vi "host-C_Exp.vi"() -> (0 "K(Indicator)":fxp<+/-,64,32>=1.52587890625e-05, 1 "degree":dbl=0.1952712924057206, 2 "Nominal Freq":fxp<+/-,64,32>=0.494873046875)   [LabVIEW 2012]
uses:
  <vilib>/FPGAPlugInAG/PCI-7831R/niLvFpga_Open_PCI-7831R.vi
  <vilib>/Utility/error.llb/Error Cluster From Error Code.vi
  <vilib>/rvi/errors/niLvFpgaAdjustHostInterfaceError.vi
  <vilib>/FPGAPlugInAG/PCI-7831R/niLvFpga_Run_PCI-7831R.vi
  <vilib>/FPGAPlugInAG/PCI-7831R/niLvFpga_Abort_PCI-7831R.vi
  <vilib>/FPGAPlugInAG/PCI-7831R/niLvFpga_Close_PCI-7831R.vi
  <vilib>/rvi/interface/common/dynamic/niFpgaDynamicAddResources.vi
  <vilib>/FPGAPlugInAG/Dynamic/niLvFpga_Abort_Dynamic.vi
  <vilib>/FPGAPlugInAG/Dynamic/niLvFpga_Close_Dynamic.vi
  <vilib>/Utility/file.llb/Write To Spreadsheet File (DBL).vi
  <vilib>/rvi/interface/nirviOpenFPGA/nirviOpenFPGA.xnode
  SB130-XPS/Documents/FPGA-project-apporach-retraction/FPGA Bitfiles/Apporach-Retract_FPGATarget_LIAFPGA3a-PDTest_L-X5ia9B-g4.lvbitx
  LIA_FPGA3a-PD Test.vi
  <vilib>/rvi/interface/nirviReadWriteControl/nirviReadWriteControl.xnode
  <vilib>/rvi/interface/nirviMethod/nirviMethod.xnode
  <vilib>/rvi/interface/nirviCloseFPGA/nirviCloseFPGA.xnode
  NiFpgaLv.dll
  <vilib>/rvi/interface/Simulation/niFpgaSimulationCallBeginRW.vi
panel:
  in  "Path 5":path
  in  "name-file 11":string="approach-15a"
  out "String 11":string
  in  "Path 7":path
  in  "name-file 9":string="approach-15a"
  out "String 9":string
  out "P+I Error":dbl
  in  "Integral Gain":dbl
  in  "Proportional Gain":ext
  out "Setpoint":dbl
  in  "Path 4":path
  in  "name-file 4":string="approach-15a"
  out "String 4":string
  in  "Path 3":path
  in  "name-file 3":string="approach-15a"
  out "String 3":string
  in  "Path 2":path
  in  "name-file 2":string="approach-15a"
  out "String 2":string
  in  "Data Collector":bool
  out "String":string
  in  "name-file":string="approach-15a"
  in  "Path":path
  out "Standardized nominal freq":dbl
  in  "Delta Nominal Frequency":dbl
  out "Ref":i32
  out "Sig":i32
  out "Sin":dbl(graph)
  out "Phase":dbl
  out "Ze Output":dbl=2.3841857910156248e-12
  out "The Decs":dbl=7.8125e-09
  out "LSB Weight":dbl=0.00030517578125
  in  "K":fxp<+,16,0>=1.52587890625e-05
  in  "nominal freq 2":fxp<+,16,0>=0.494873046875
  out "x*y":dbl=0.015
  in  "stop 2":bool
  out "3rd stages":i32=1
  out "3rd decimation":i32=977
  out "1st decimation":i32=1
  out "2nd decimation":i32=128
  in  "Time Constant [s]":dbl=2.5 min=0.0 step=0.0001 format="%.2f"
  in  "Filter Rolloff":enum16{"20 dB", "40 dB", "60 dB", "80 dB"}(ring)
  out "Actual Sampling Frequency":dbl=200000.0
  in  "input range of 9205":dbl=10.0
  in  "Sampling Frequency":dbl=200000.0 min=1000.0 max=250000.0
  in  "stop":bool
  out "r":dbl(graph)=0.5098420210496609
  out "y":dbl=0.0017376029872894286
  out "x":dbl=0.5098390600609779
  out "f":dbl(graph)=31000.332441180944
  in  "dec2":i16=1
  in  "nominal freq":dbl=30000.0 min=500.0 max=125000.0
  in  "dec1":i16=1000
  in  "stages":i8=1 min=1 max=2
  in  "decimation":i16=1000
  # "Sampling Frequency"
  # "CIC First Decimation"
  # "MA Stages"
  # "CIC Second Decimation"
  # "PLL Nominal Frequency"
  # "MA Decimation"
  # "PLL Frequency Output"
  # "LIA Output"
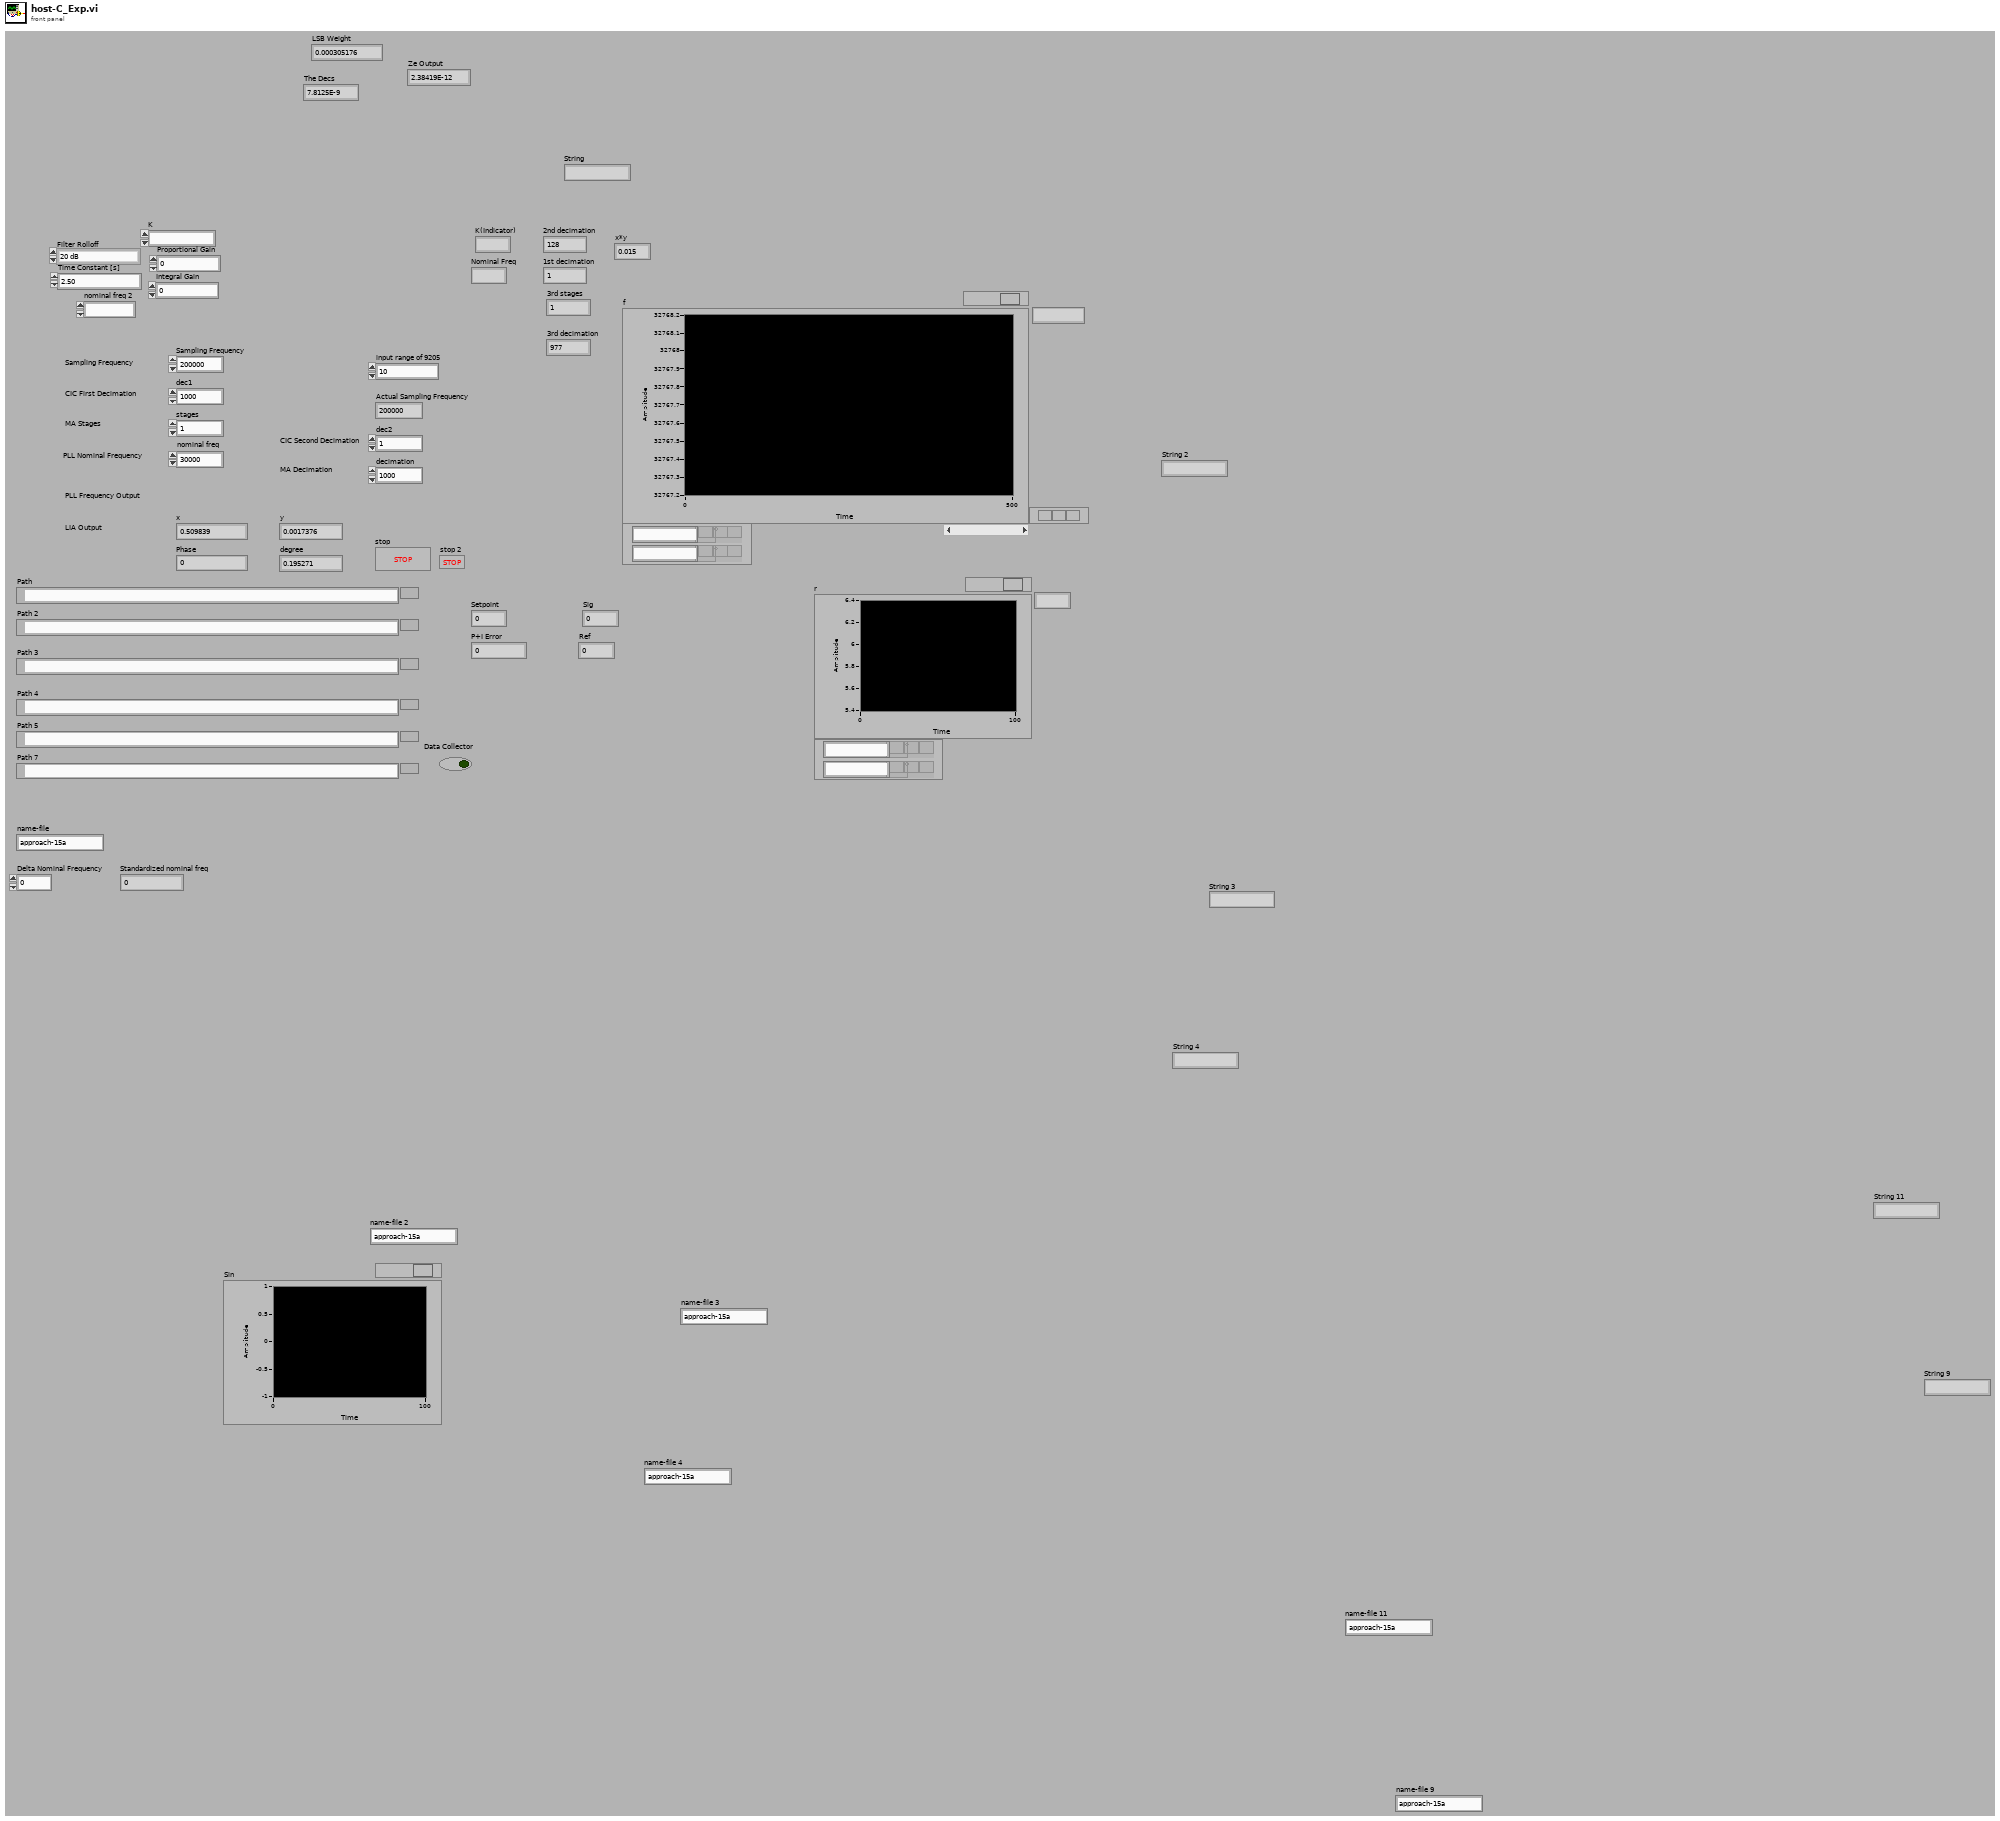
[diagram p1: front panel]
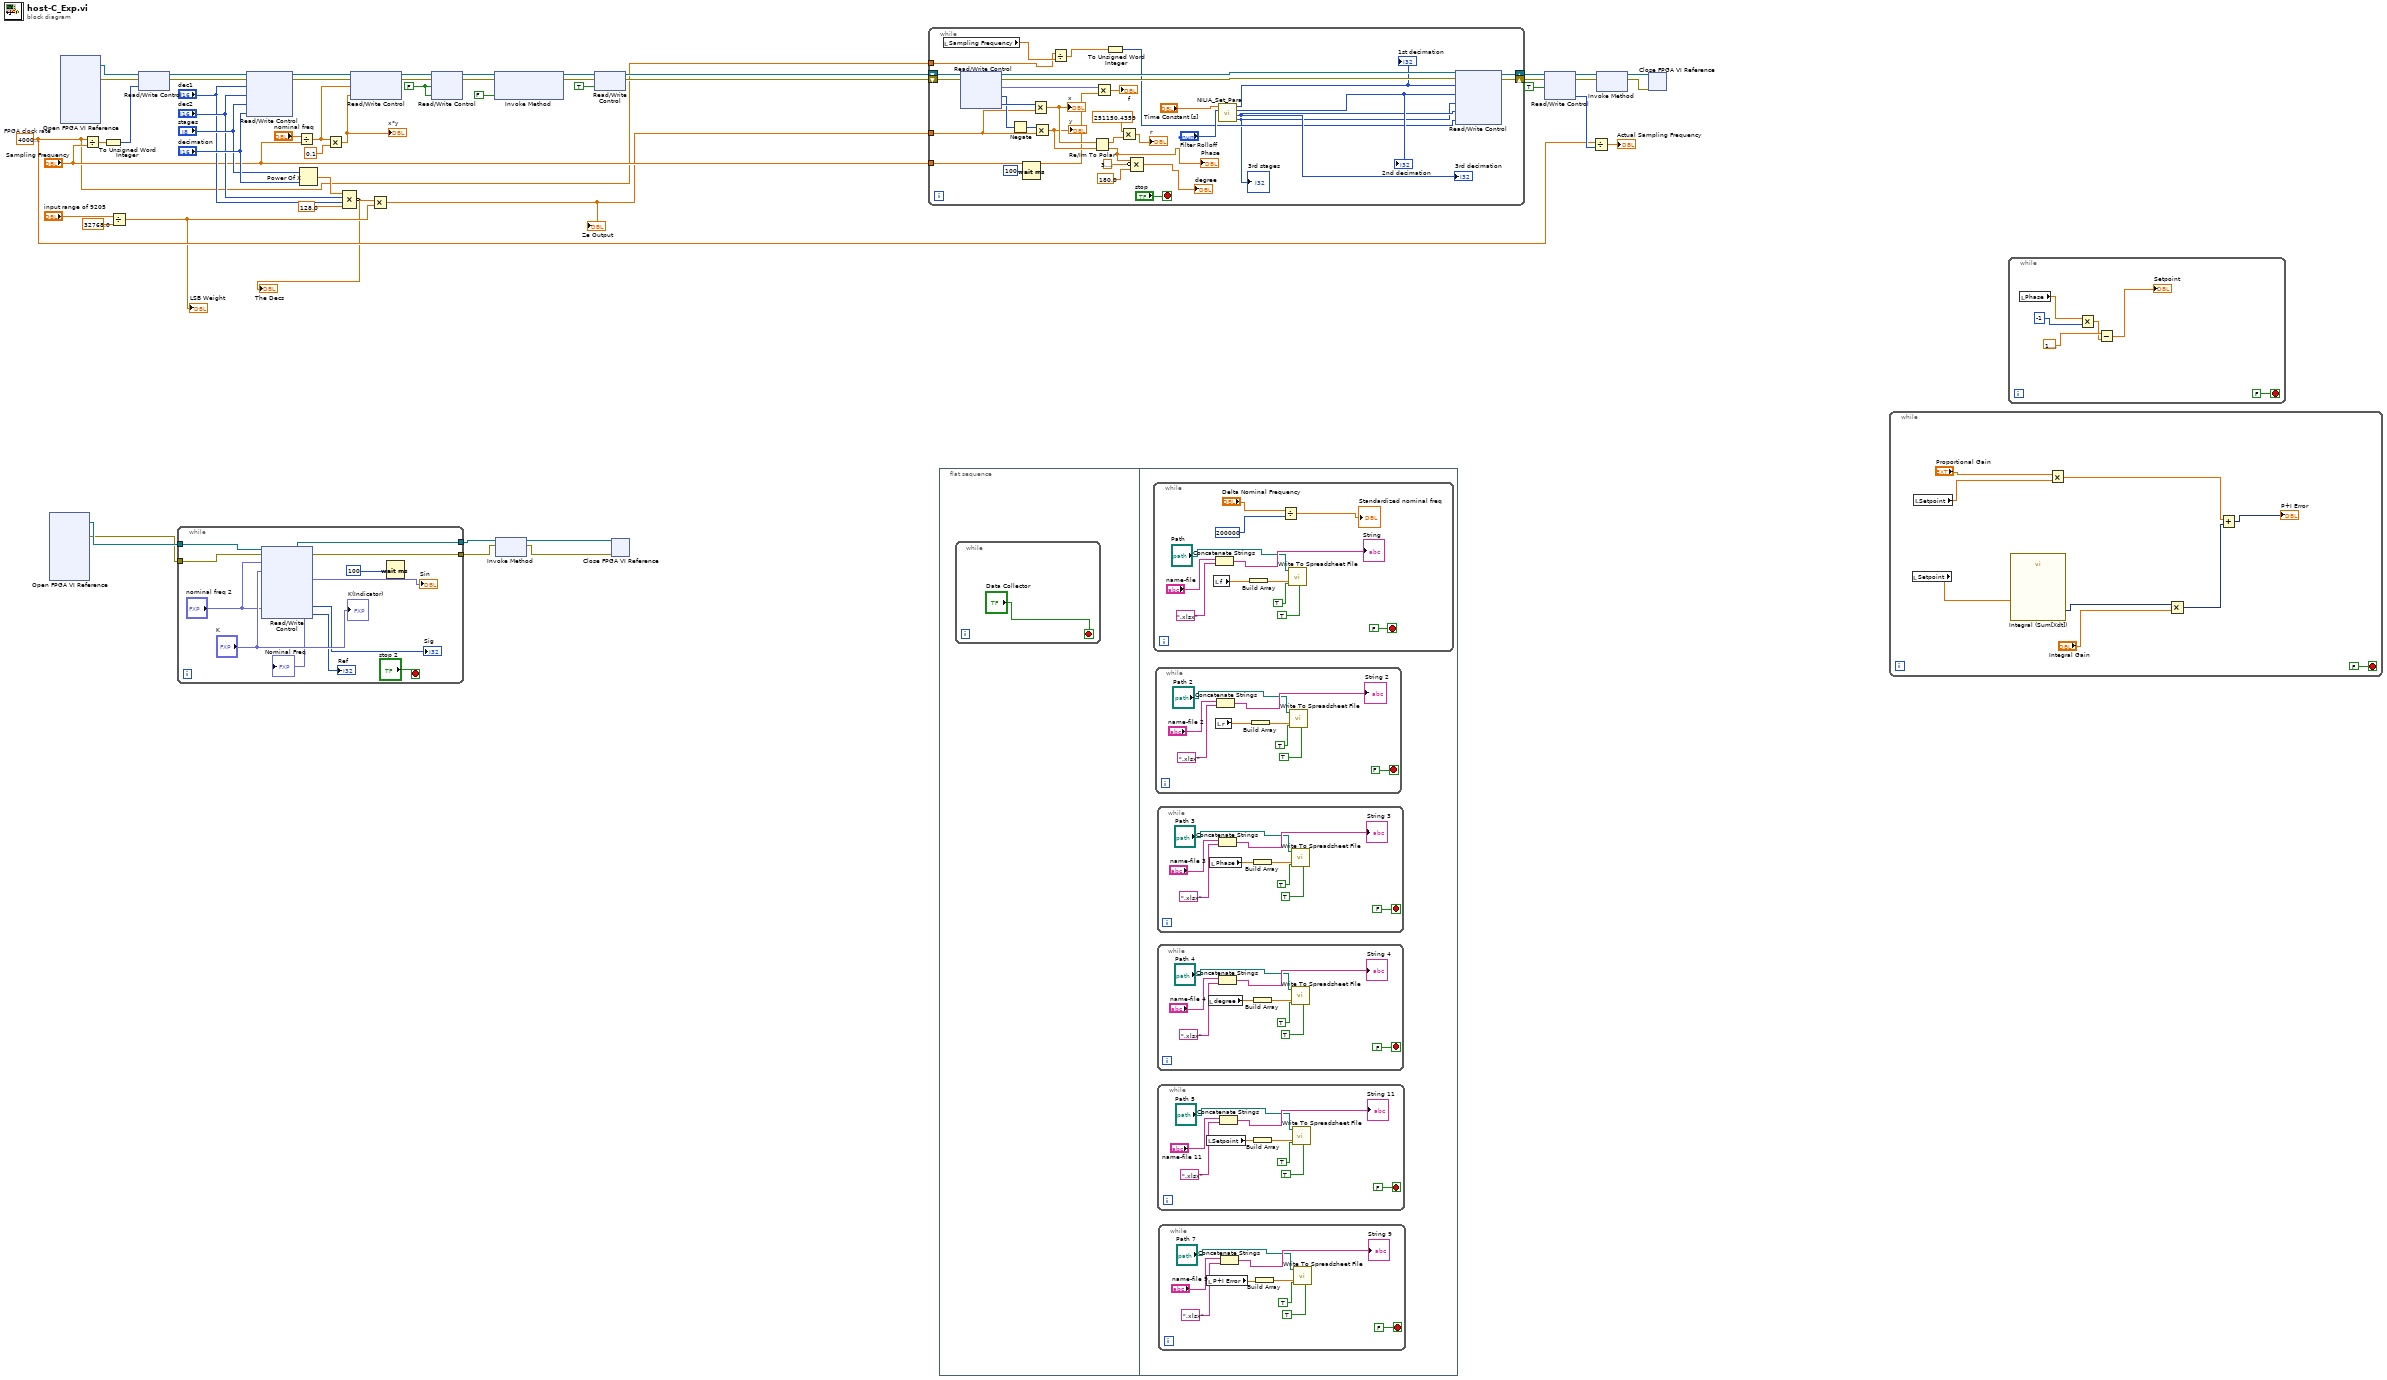
[diagram p0: block diagram]
diagram:
  w13 = 40000000.0  # FPGA clock rate
  w30 = FALSE ("start")
  n1 = xnode "Open FPGA VI Reference"() -> ("FPGA VI Reference Out"=w2:refnum<k20>, "error out"=w1:errorcluster)  [unwired: 2 in]
  n2 = xnode "Open FPGA VI Reference"() -> ("FPGA VI Reference Out"=w3:refnum<k20>, "error out"=w4:errorcluster)  [unwired: 2 in]
  n3 = Divide(x=w13, y="Sampling Frequency") -> (x/y=w23:dbl)
  n4 = To Unsigned Word Integer(number=w23) -> (unsigned 16bit integer=w22:u16)
  n5 = Divide(x="input range of 9205", y=32768.0) -> (x/y=w7:dbl)
  "LSB Weight" <- w7
  n6 = xnode "Read/Write Control"("FPGA VI Reference In"=w3, "error in"=w4, "Period"=w22) -> ("FPGA VI Reference Out"=w25:refnum<k20>, "error out"=w24:errorcluster)
  n7 = while {
    tunnel: w2 -> [w52]
    tunnel: w1 -> [w61]
    tunnel: [w60] -> w12
    tunnel: [w59] -> w11
    stop <- "stop 2" stop-if-true
    n8 = xnode "Read/Write Control"("FPGA VI Reference In"=w52, "error in"=w61, "nominal freq"="nominal freq 2", "K"="K") -> ("FPGA VI Reference Out"=w60:refnum<k20>, "error out"=w59:errorcluster, "Sin"=→"Sin":fxp<+/-,14,2>, "sig"=→"Sig":i16, "ref"=→"Ref":i16)  [unwired: 2 out]
    n9 = Wait (ms)(milliseconds to wait=u32 100) -> ()  [unwired: 1 out]
    "K(Indicator)" <- "K"
    "Nominal Freq" <- "nominal freq 2"
  }
  n10 = xnode "Read/Write Control"("FPGA VI Reference In"=w25, "error in"=w24, "dec1"="dec1", "dec2"="dec2", "stages"="stages", "decimation"="decimation") -> ("FPGA VI Reference Out"=w51:refnum<k20>, "error out"=w50:errorcluster)
  n11 = Divide(x="nominal freq", y="Sampling Frequency") -> (x/y=w19:dbl)
  n12 = Power Of X(1:"decimation", 2:"stages") -> (0:w46:dbl)
  n13 = Multiply(x=w19, y=0.1) -> (x*y=w8:dbl)
  "x*y" <- w8
  n14 = Compound Arithmetic op=MULTIPLY(w46, "dec2", "dec1", 128.0) -> (invert w6:dbl)
  "The Decs" <- w6
  n15 = xnode "Read/Write Control"("FPGA VI Reference In"=w51, "error in"=w50, "nominal freq"=w19, "K"=w8) -> ("FPGA VI Reference Out"=w34:refnum<k20>, "error out"=w33:errorcluster)
  n16 = Multiply(x=w6, y=w7) -> (x*y=w5:dbl)
  "Ze Output" <- w5
  n17 = xnode "Read/Write Control"("FPGA VI Reference In"=w34, "error in"=w33, "start"=w30, "stop"=w30) -> ("FPGA VI Reference Out"=w32:refnum<k20>, "error out"=w31:errorcluster)
  n18 = xnode "Invoke Method"("FPGA VI Reference In"=w32, "error in"=w31, "Wait Until Done (F)"=FALSE) -> ("FPGA VI Reference Out"=w39:refnum<k20>, "error out"=w37:errorcluster)
  n19 = xnode "Invoke Method"("FPGA VI Reference In"=w12, "error in"=w11) -> ("FPGA VI Reference Out"=w10:refnum<k20>, "error out"=w9:errorcluster)
  n20 = xnode "Read/Write Control"("FPGA VI Reference In"=w39, "error in"=w37, "start"=TRUE) -> ("FPGA VI Reference Out"=w38:refnum<k20>, "error out"=w36:errorcluster)
  n21 = xnode "Close FPGA VI Reference"("FPGA VI Reference In"=w10, "error in"=w9) -> ()  [unwired: 1 out]
  n22 = while {
    shift-right: [w79] -> w42
    shift-left: w38 -> [w94]
    shift-right: [w78] -> w41
    shift-left: w36 -> [w93]
    tunnel: w5 -> [w90]
    tunnel: "Sampling Frequency" -> [w82]
    tunnel: w13 -> [w71]
    stop <- "stop" stop-if-true
    n23 = local read "Sampling Frequency"() -> (w72:dbl)
    n24 = xnode "Read/Write Control"("FPGA VI Reference In"=w94, "error in"=w93) -> ("FPGA VI Reference Out"=w79:refnum<k20>, "error out"=w78:errorcluster, "f"=w83:fxp<+/-,32,0>, "channelQ"=w91:i64, "channelI"=w92:i64)
    n25 = Negate(x=w91) -> (-x=w80:i64)
    n26 = Wait (ms)(milliseconds to wait=u32 100) -> ()  [unwired: 1 out]
    n27 = Multiply(x=w92, y=w90) -> (x*y=w89:dbl)
    "x" <- w89
    n28 = Multiply(x=w80, y=w90) -> (x*y=w88:dbl)
    "y" <- w88
    n29 = Divide(x=w71, y=w72) -> (x/y=w70:dbl)
    n30 = Re/Im To Polar(2:w88, 3:w89) -> (0:w63:dbl, 1:w66:dbl)
    "Phase" <- w63
    n31 = Multiply(x=w83, y=w82) -> (x*y=→"f":dbl)
    n32 = To Unsigned Word Integer(number=w70) -> (unsigned 16bit integer=w69:u16)
    n33 = Multiply(x=251150.4359, y=w66) -> (x*y=→"r":dbl)
    n34 = Compound Arithmetic op=MULTIPLY(w63, invert 3.141592653589793, 180.0 ("value")) -> (→"degree":dbl)
    n35 = call "NILIA_Set_Para.vi"("rolloff"="Filter Rolloff", "TC [sec]"="Time Constant [s]") -> ("3rd stages"=w68:i32, "3rd decimation"=w73:i32, "2nd decimation"=w74:i32, "1st decimation"=w75:i32)  [unwired: 5 in, 1 out]
    "2nd decimation" <- w74
    "1st decimation" <- w75
    "3rd decimation" <- w73
    "3rd stages" <- w68
    n36 = xnode "Read/Write Control"("FPGA VI Reference In"=w79, "error in"=w78, "dec1"=w75, "dec2"=w74, "stages"=w68, "decimation"=w73, "Period"=w69) -> ()  [unwired: 2 out]
  }
  n37 = flat-sequence {
    frame #0 {
      n38 = while {
        stop <- "Data Collector" stop-if-true
      }
    }
    frame #1 {
      n39 = while {
        stop <- FALSE stop-if-true
        n40 = local read "f"() -> (w148:dbl)
        n41 = Concatenate Strings("name-file", ".xlsx") -> (→"String":string)
        n42 = Build Array(w148) -> (w147:dbl[])
        n43 = Divide(x="Delta Nominal Frequency", y=200000) -> (x/y=→"Standardized nominal freq":dbl)
        n44 = call-poly <vilib>:"Write To Spreadsheet File.vi"("transpose? (no:F)"=TRUE, "append to file? (new file:F)"=TRUE, "1D data"=w147, "file path (dialog if empty)"="Path") -> ()  [unwired: 4 in, 1 out]
      }
      n45 = while {
        stop <- FALSE stop-if-true
        n46 = local read "r"() -> (w139:dbl)
        n47 = Concatenate Strings("name-file 2", ".xlsx") -> (→"String 2":string)
        n48 = Build Array(w139) -> (w138:dbl[])
        n49 = call-poly <vilib>:"Write To Spreadsheet File.vi"("transpose? (no:F)"=TRUE, "append to file? (new file:F)"=TRUE, "1D data"=w138, "file path (dialog if empty)"="Path 2") -> ()  [unwired: 4 in, 1 out]
      }
      n50 = while {
        stop <- FALSE stop-if-true
        n51 = local read "Phase"() -> (w130:dbl)
        n52 = Concatenate Strings("name-file 3", ".xlsx") -> (→"String 3":string)
        n53 = Build Array(w130) -> (w129:dbl[])
        n54 = call-poly <vilib>:"Write To Spreadsheet File.vi"("transpose? (no:F)"=TRUE, "append to file? (new file:F)"=TRUE, "1D data"=w129, "file path (dialog if empty)"="Path 3") -> ()  [unwired: 4 in, 1 out]
      }
      n55 = while {
        stop <- FALSE stop-if-true
        n56 = local read "degree"() -> (w121:dbl)
        n57 = Concatenate Strings("name-file 4", ".xlsx") -> (→"String 4":string)
        n58 = Build Array(w121) -> (w120:dbl[])
        n59 = call-poly <vilib>:"Write To Spreadsheet File.vi"("transpose? (no:F)"=TRUE, "append to file? (new file:F)"=TRUE, "1D data"=w120, "file path (dialog if empty)"="Path 4") -> ()  [unwired: 4 in, 1 out]
      }
      n60 = while {
        stop <- FALSE stop-if-true
        n61 = local read "Setpoint"() -> (w103:dbl)
        n62 = Concatenate Strings("name-file 11", ".xlsx") -> (→"String 11":string)
        n63 = Build Array(w103) -> (w102:dbl[])
        n64 = call-poly <vilib>:"Write To Spreadsheet File.vi"("transpose? (no:F)"=TRUE, "append to file? (new file:F)"=TRUE, "1D data"=w102, "file path (dialog if empty)"="Path 5") -> ()  [unwired: 4 in, 1 out]
      }
      n65 = while {
        stop <- FALSE stop-if-true
        n66 = local read "P+I Error"() -> (w112:dbl)
        n67 = Concatenate Strings("name-file 9", ".xlsx") -> (→"String 9":string)
        n68 = Build Array(w112) -> (w111:dbl[])
        n69 = call-poly <vilib>:"Write To Spreadsheet File.vi"("transpose? (no:F)"=TRUE, "append to file? (new file:F)"=TRUE, "1D data"=w111, "file path (dialog if empty)"="Path 7") -> ()  [unwired: 4 in, 1 out]
      }
    }
  }
  n70 = xnode "Read/Write Control"("FPGA VI Reference In"=w42, "error in"=w41, "stop"=TRUE) -> ("FPGA VI Reference Out"=w29:refnum<k20>, "error out"=w28:errorcluster, "ticks"=w15:u16)
  n71 = Divide(x=w13, y=w15) -> (x/y=→"Actual Sampling Frequency":dbl)
  n72 = xnode "Invoke Method"("FPGA VI Reference In"=w29, "error in"=w28) -> ("FPGA VI Reference Out"=w27:refnum<k20>, "error out"=w26:errorcluster)
  n73 = xnode "Close FPGA VI Reference"("FPGA VI Reference In"=w27, "error in"=w26) -> ()  [unwired: 1 out]
  n74 = while {
    stop <- FALSE stop-if-true
    n75 = local read "Setpoint"() -> (w158:dbl)
    n76 = local read "Setpoint"() -> (w160:dbl)
    n77 = call "Integral (Sum[Xdt])"("Signals"=w158) -> ("Result"=w156:dynamicdata)  [unwired: 5 in, 1 out]
    n78 = Multiply(x="Proportional Gain", y=w160) -> (x*y=w155:ext)
    n79 = Multiply(x=w156, y="Integral Gain") -> (x*y=w154:dynamicdata)
    n80 = Add(x=w155, y=w154) -> (x+y=→"P+I Error":dynamicdata)
  }
  n81 = while {
    stop <- FALSE stop-if-true
    n82 = local read "Phase"() -> (w164:dbl)
    n83 = Multiply(x=w164, y=-1) -> (x*y=w162:dbl)
    n84 = Subtract(x=1.5707963267948966, y=w162) -> (x-y=→"Setpoint":dbl)
  }
